vi "Remove Units Panel 2.vi"(0 "System#":u8, 7 "Rack Number":i8=2 min=1 max=16, 8 "AutoAge.ini  File Path":path=path "\\\\Beco\\autoage/config/autoage.ini") -> ()   [LabVIEW 2021]
uses:
  Main Controls System v8.0/AutoAge Globals.vi
panel:
  in  "Update":bool
  in  "Row33 to 40":bool
  in  "Row25 to 32":bool
  in  "Row17 to 24":bool
  in  "Row9 to 16":bool
  in  "Row1 to 8":bool
  in  "Select All":bool
  in  "40":bool
  in  "39":bool
  in  "38":bool
  in  "37":bool
  in  "36":bool
  in  "35":bool
  in  "34":bool
  in  "33":bool
  in  "32":bool
  in  "31":bool
  in  "30":bool
  in  "29":bool
  in  "28":bool
  in  "27":bool
  in  "26":bool
  in  "25":bool
  in  "24":bool
  in  "23":bool
  in  "22":bool
  in  "21":bool
  in  "20":bool
  in  "19":bool
  in  "18":bool
  in  "17":bool
  in  "16":bool
  in  "15":bool
  in  "14":bool
  in  "13":bool
  in  "12":bool
  in  "11":bool
  in  "10":bool
  in  "9":bool
  in  "8":bool
  in  "7":bool
  in  "6":bool
  in  "5":bool
  in  "4":bool
  in  "3":bool
  in  "2":bool
  in  "1":bool
  out "Rack":i8=1 min=1 max=16
  in  "Done":bool
  # "Click to Remove active positions.  A red square in a position indicates that a position is going to run."
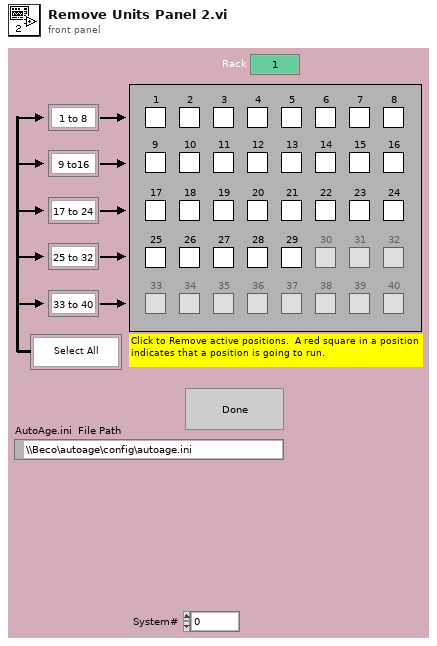
[diagram p1: front panel]
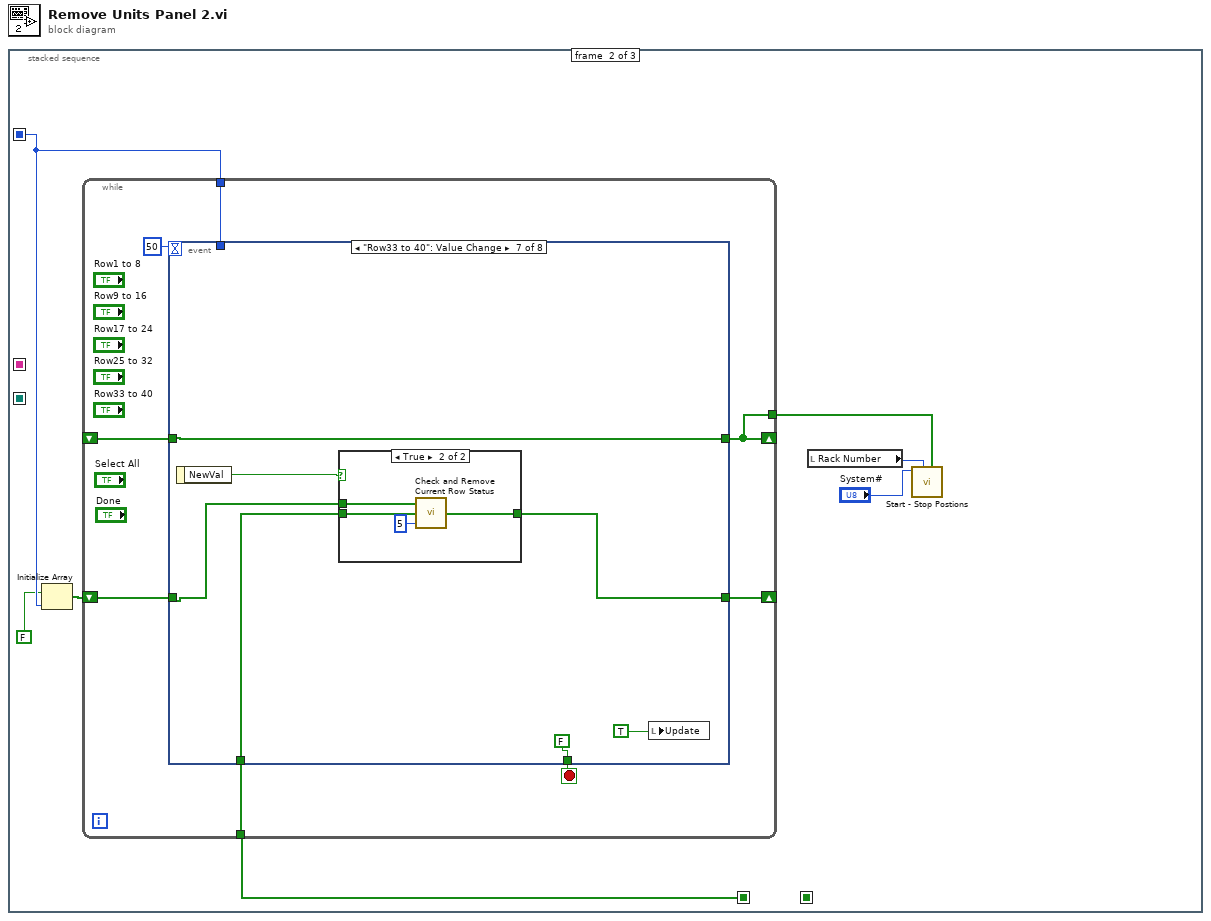
[diagram p0: block diagram]
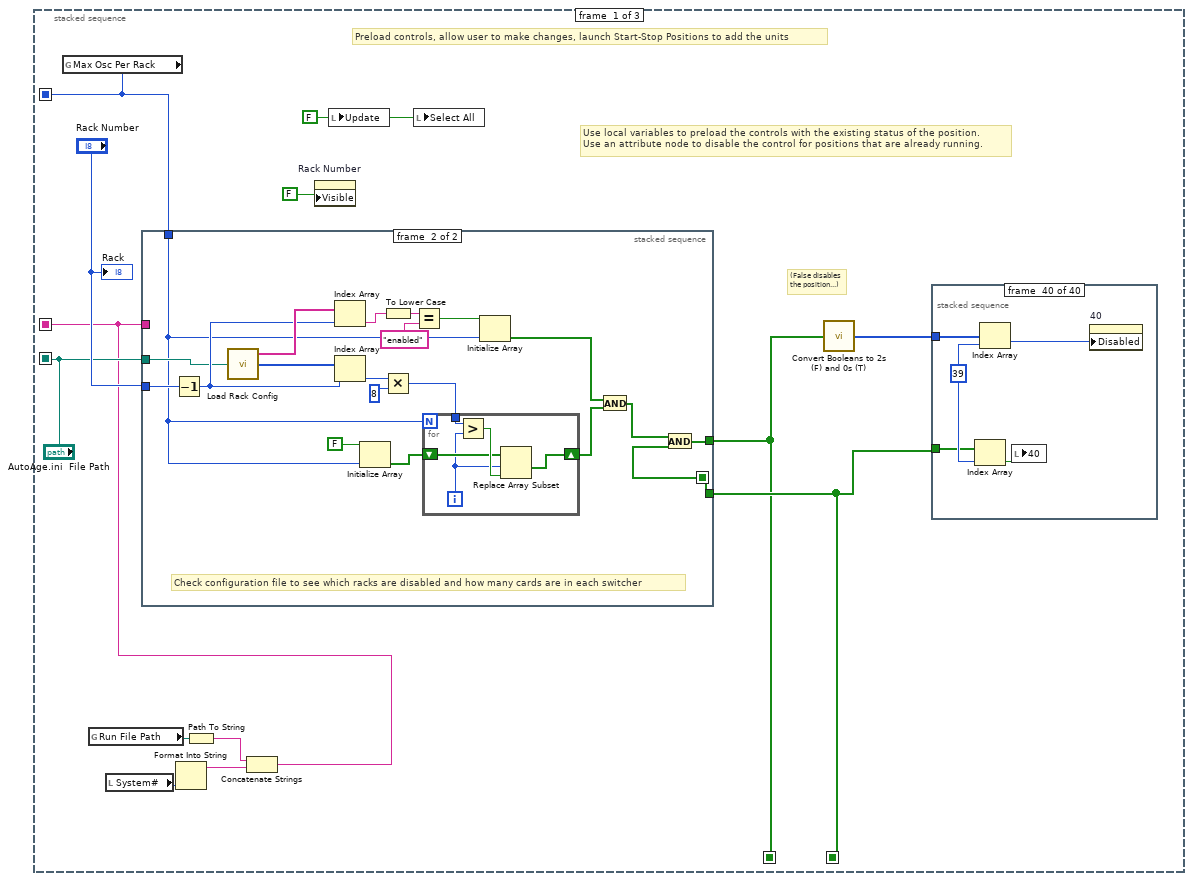
[diagram p2: hidden frame]
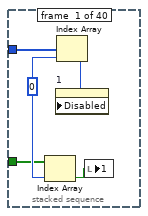
[diagram p3: hidden frame]
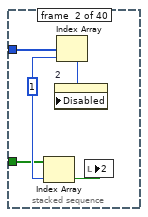
[diagram p4: hidden frame]
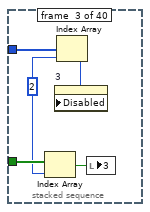
[diagram p5: hidden frame]
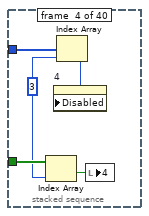
[diagram p6: hidden frame]
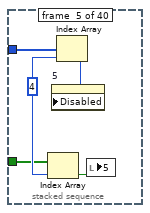
[diagram p7: hidden frame]
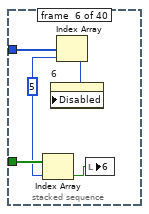
[diagram p8: hidden frame]
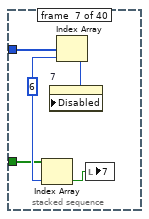
[diagram p9: hidden frame]
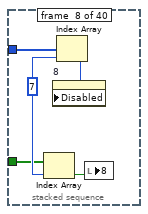
[diagram p10: hidden frame]
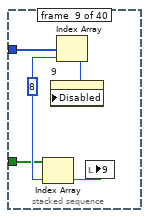
[diagram p11: hidden frame]
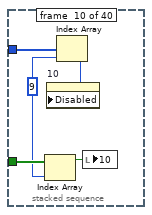
[diagram p12: hidden frame]
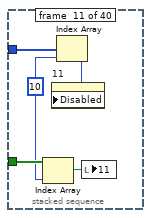
[diagram p13: hidden frame]
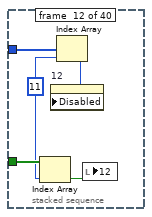
[diagram p14: hidden frame]
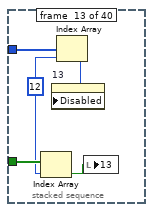
[diagram p15: hidden frame]
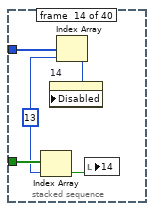
[diagram p16: hidden frame]
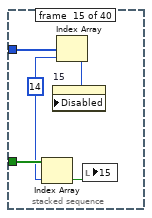
[diagram p17: hidden frame]
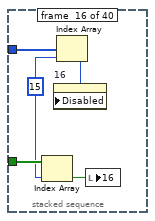
[diagram p18: hidden frame]
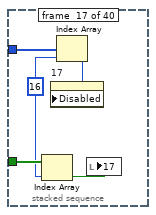
[diagram p19: hidden frame]
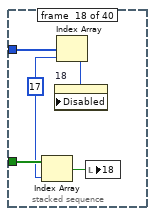
[diagram p20: hidden frame]
diagram:
  n1 = stacked-sequence {
    seq-local: [w10 _ _] -> [_ _ _]
    seq-local: [w9 _ _] -> [_ w267 _]
    seq-local: [w7 _ _] -> [_ w266 _]
    seq-local: ["AutoAge.ini  File Path" _ _] -> [_ _ _]
    seq-local: [w1 _ _] -> [_ _ _]
    frame #0 {
      w8 = FALSE ("Update")
      # "(False disables\nthe position...)"
      # "Preload controls, allow user to make changes, launch Start-Stop Positions to add the units"
      # "Use local variables to preload the controls with the existing status of the position.\nUse an attribute node to disable the control for positions that are already running."
      n2 = global read "AutoAge Globals.vi" "Max Osc Per Rack"() -> (w7:u16)
      n3 = global read "AutoAge Globals.vi" "Run File Path"() -> (w3:path)
      n4 = local read "System#"() -> (w4:u8)
      n5 = Format Into String(w4) -> (resulting string=w6:string)  [unwired: 3 in, 1 out]
      n6 = Path To String(path=w3) -> (string=w5:string)
      n7 = Concatenate Strings(w5, w6) -> (w1:string)
      n8 = stacked-sequence {
        seq-local: [w217 _] -> [_ w242]
        tunnel: "Rack Number" -> [w216 w250]
        tunnel: [_ w241] -> w9
        tunnel: [_ w242] -> w10
        tunnel: "AutoAge.ini  File Path" -> [_ w239]
        tunnel: w1 -> [w215 _]
        tunnel: w7 -> [w214 w238]
        frame #0 {
          # "Scan the disk to see which positions are currently running"
          n9 = for {
            N: w214 -> [_]
            tunnel: [w235] -> w217 mode=indexing
            tunnel: w216 -> [w223]
            tunnel: w215 -> [w220]
            i -> [w236]
            w221 = "-"
            n10 = Increment(x=w236) -> (x+1=w224:i32)
            n11 = Number To Decimal String(number=w223) -> (decimal integer string=w227:string)  [unwired: 1 in]
            n12 = Number To Decimal String(number=w224) -> (decimal integer string=w226:string)  [unwired: 1 in]
            n13 = Concatenate Strings(w220, w221, w227, w221, w226, ".run") -> (w225:string)
            n14 = String To Path(string=w225) -> (path=w234:path)
            n15 = Open/Create/Replace File(file path (use dialog)=w234, access (0:read/write)=1) -> (refnum out=w218:refnum<file>, error out=w219:errorcluster)  [unwired: 4 in, 1 out]
            n16 = Deny Access(4:w219, 6:1, 7:w218) -> (0:w231:errorcluster, 3:w228:refnum<file>)
            n17 = Close File(refnum=w228) -> ()  [unwired: 1 in, 2 out]
            n18 = Unbundle(w231) -> ("code"=w229:i32)  [unwired: 2 out]
            n19 = Equal?(x=w229, y=0) -> (x = y?=w235:bool)
          }
        }
        frame #1 {
          # "Check configuration file to see which racks are disabled and how many cards are in each switcher"
          n20 = Decrement(x=w250) -> (x-1=w240:i8)
          n21 = call "Load Rack Config"("AutoAge.ini  File Path"=w239) -> ("Rack Status"=w251:string[], "# of Cards"=w255:i32[])  [unwired: 1 out]
          n22 = Index Array(array=w251, index=w240) -> (element=w249:string)
          n23 = Index Array(array=w255, index=w240) -> (element=w256:i32)
          n24 = Initialize Array(FALSE, w238) -> (w245:bool[])
          n25 = To Lower Case(string=w249) -> (all lower case string=w254:string)
          n26 = Multiply(x=w256, y=8) -> (x*y=w246:i32)
          n27 = Equal?(x=w254, y="enabled") -> (x = y?=w248:bool)
          n28 = for {
            N: w238 -> [_]
            tunnel: w246 -> [w261]
            shift-right: [w258] -> w243
            shift-left: w245 -> [w259]
            i -> [w257]
            n29 = Greater?(x=w261, y=w257) -> (0:w260:bool)
            n30 = Replace Array Subset(array=w259, new element=w260, index=w257) -> (w258:bool[])
          }
          n31 = Initialize Array(w248, w238) -> (w244:bool[])
          n32 = And(x=w244, y=w243) -> (x .and. y?=w237:bool[])
          n33 = And(x=w237, y=w242) -> (x .and. y?=w241:bool[])
        }
      }
      n34 = property on="Rack Number" class="DigNum (strict)"("Visible"=FALSE) -> ()  [unwired: 2 in, 2 out]
      n35 = local write "Update"(w8) -> ()
      n36 = local write "Select All"(w8) -> ()
      n37 = call "Convert Booleans to 2s (F) and 0s (T)"("Boolean Array"=w9) -> ("2s and 0s"=w11:i8[])
      n38 = stacked-sequence {
        tunnel: w11 -> [w18 w23 w28 w33 w38 w43 w48 w53 w58 w63 w68 w73 w78 w83 w88 w93 w98 w103 w108 w113 w118 w123 w128 w133 w138 w143 w148 w153 w158 w163 w168 w173 w178 w183 w188 w193 w198 w203 w208 w213]
        tunnel: w10 -> [w15 w20 w27 w32 w36 w42 w46 w51 w56 w62 w67 w72 w77 w82 w87 w92 w97 w102 w107 w112 w117 w122 w127 w132 w137 w142 w147 w152 w157 w162 w167 w172 w177 w182 w187 w192 w197 w202 w207 w210]
        frame #0 {
          w16 = 0
          n39 = Index Array(array=w15, index=w16) -> (element=w17:bool)
          n40 = Index Array(array=w18, index=w16) -> (element=w14:i8)
          n41 = property on="1" class="Bool (strict)"("Disabled"=w14) -> ()  [unwired: 2 in, 2 out]
          n42 = local write "1"(w17) -> ()
        }
        frame #1 {
          w22 = 1
          n43 = Index Array(array=w20, index=w22) -> (element=w21:bool)
          n44 = Index Array(array=w23, index=w22) -> (element=w19:i8)
          n45 = property on="2" class="Bool (strict)"("Disabled"=w19) -> ()  [unwired: 2 in, 2 out]
          n46 = local write "2"(w21) -> ()
        }
        frame #2 {
          w26 = 2
          n47 = Index Array(array=w27, index=w26) -> (element=w25:bool)
          n48 = Index Array(array=w28, index=w26) -> (element=w24:i8)
          n49 = property on="3" class="Bool (strict)"("Disabled"=w24) -> ()  [unwired: 2 in, 2 out]
          n50 = local write "3"(w25) -> ()
        }
        frame #3 {
          w31 = 3
          n51 = Index Array(array=w32, index=w31) -> (element=w30:bool)
          n52 = Index Array(array=w33, index=w31) -> (element=w29:i8)
          n53 = property on="4" class="Bool (strict)"("Disabled"=w29) -> ()  [unwired: 2 in, 2 out]
          n54 = local write "4"(w30) -> ()
        }
        frame #4 {
          w37 = 4
          n55 = Index Array(array=w36, index=w37) -> (element=w35:bool)
          n56 = Index Array(array=w38, index=w37) -> (element=w34:i8)
          n57 = property on="5" class="Bool (strict)"("Disabled"=w34) -> ()  [unwired: 2 in, 2 out]
          n58 = local write "5"(w35) -> ()
        }
        frame #5 {
          w41 = 5
          n59 = Index Array(array=w42, index=w41) -> (element=w40:bool)
          n60 = Index Array(array=w43, index=w41) -> (element=w39:i8)
          n61 = property on="6" class="Bool (strict)"("Disabled"=w39) -> ()  [unwired: 2 in, 2 out]
          n62 = local write "6"(w40) -> ()
        }
        frame #6 {
          w47 = 6
          n63 = Index Array(array=w46, index=w47) -> (element=w45:bool)
          n64 = Index Array(array=w48, index=w47) -> (element=w44:i8)
          n65 = property on="7" class="Bool (strict)"("Disabled"=w44) -> ()  [unwired: 2 in, 2 out]
          n66 = local write "7"(w45) -> ()
        }
        frame #7 {
          w52 = 7
          n67 = Index Array(array=w51, index=w52) -> (element=w50:bool)
          n68 = Index Array(array=w53, index=w52) -> (element=w49:i8)
          n69 = property on="8" class="Bool (strict)"("Disabled"=w49) -> ()  [unwired: 2 in, 2 out]
          n70 = local write "8"(w50) -> ()
        }
        frame #8 {
          w57 = 8
          n71 = Index Array(array=w56, index=w57) -> (element=w55:bool)
          n72 = Index Array(array=w58, index=w57) -> (element=w54:i8)
          n73 = property on="9" class="Bool (strict)"("Disabled"=w54) -> ()  [unwired: 2 in, 2 out]
          n74 = local write "9"(w55) -> ()
        }
        frame #9 {
          w60 = 9
          n75 = Index Array(array=w62, index=w60) -> (element=w61:bool)
          n76 = Index Array(array=w63, index=w60) -> (element=w59:i8)
          n77 = property on="10" class="Bool (strict)"("Disabled"=w59) -> ()  [unwired: 2 in, 2 out]
          n78 = local write "10"(w61) -> ()
        }
        frame #10 {
          w65 = 10
          n79 = Index Array(array=w67, index=w65) -> (element=w66:bool)
          n80 = Index Array(array=w68, index=w65) -> (element=w64:i8)
          n81 = property on="11" class="Bool (strict)"("Disabled"=w64) -> ()  [unwired: 2 in, 2 out]
          n82 = local write "11"(w66) -> ()
        }
        frame #11 {
          w70 = 11
          n83 = Index Array(array=w72, index=w70) -> (element=w71:bool)
          n84 = Index Array(array=w73, index=w70) -> (element=w69:i8)
          n85 = property on="12" class="Bool (strict)"("Disabled"=w69) -> ()  [unwired: 2 in, 2 out]
          n86 = local write "12"(w71) -> ()
        }
        frame #12 {
          w75 = 12
          n87 = Index Array(array=w77, index=w75) -> (element=w76:bool)
          n88 = Index Array(array=w78, index=w75) -> (element=w74:i8)
          n89 = property on="13" class="Bool (strict)"("Disabled"=w74) -> ()  [unwired: 2 in, 2 out]
          n90 = local write "13"(w76) -> ()
        }
        frame #13 {
          w81 = 13
          n91 = Index Array(array=w82, index=w81) -> (element=w80:bool)
          n92 = Index Array(array=w83, index=w81) -> (element=w79:i8)
          n93 = property on="14" class="Bool (strict)"("Disabled"=w79) -> ()  [unwired: 2 in, 2 out]
          n94 = local write "14"(w80) -> ()
        }
        frame #14 {
          w86 = 14
          n95 = Index Array(array=w87, index=w86) -> (element=w85:bool)
          n96 = Index Array(array=w88, index=w86) -> (element=w84:i8)
          n97 = property on="15" class="Bool (strict)"("Disabled"=w84) -> ()  [unwired: 2 in, 2 out]
          n98 = local write "15"(w85) -> ()
        }
        frame #15 {
          w91 = 15
          n99 = Index Array(array=w92, index=w91) -> (element=w90:bool)
          n100 = Index Array(array=w93, index=w91) -> (element=w89:i8)
          n101 = property on="16" class="Bool (strict)"("Disabled"=w89) -> ()  [unwired: 2 in, 2 out]
          n102 = local write "16"(w90) -> ()
        }
        frame #16 {
          w96 = 16
          n103 = Index Array(array=w97, index=w96) -> (element=w95:bool)
          n104 = Index Array(array=w98, index=w96) -> (element=w94:i8)
          n105 = property on="17" class="Bool (strict)"("Disabled"=w94) -> ()  [unwired: 2 in, 2 out]
          n106 = local write "17"(w95) -> ()
        }
        frame #17 {
          w101 = 17
          n107 = Index Array(array=w102, index=w101) -> (element=w100:bool)
          n108 = Index Array(array=w103, index=w101) -> (element=w99:i8)
          n109 = property on="18" class="Bool (strict)"("Disabled"=w99) -> ()  [unwired: 2 in, 2 out]
          n110 = local write "18"(w100) -> ()
        }
        frame #18 {
          w106 = 18
          n111 = Index Array(array=w107, index=w106) -> (element=w105:bool)
          n112 = Index Array(array=w108, index=w106) -> (element=w104:i8)
          n113 = property on="19" class="Bool (strict)"("Disabled"=w104) -> ()  [unwired: 2 in, 2 out]
          n114 = local write "19"(w105) -> ()
        }
        frame #19 {
          w111 = 19
          n115 = Index Array(array=w112, index=w111) -> (element=w110:bool)
          n116 = Index Array(array=w113, index=w111) -> (element=w109:i8)
          n117 = property on="20" class="Bool (strict)"("Disabled"=w109) -> ()  [unwired: 2 in, 2 out]
          n118 = local write "20"(w110) -> ()
        }
        frame #20 {
          w115 = 20
          n119 = Index Array(array=w117, index=w115) -> (element=w116:bool)
          n120 = Index Array(array=w118, index=w115) -> (element=w114:i8)
          n121 = property on="21" class="Bool (strict)"("Disabled"=w114) -> ()  [unwired: 2 in, 2 out]
          n122 = local write "21"(w116) -> ()
        }
        frame #21 {
          w121 = 21
          n123 = Index Array(array=w122, index=w121) -> (element=w120:bool)
          n124 = Index Array(array=w123, index=w121) -> (element=w119:i8)
          n125 = property on="22" class="Bool (strict)"("Disabled"=w119) -> ()  [unwired: 2 in, 2 out]
          n126 = local write "22"(w120) -> ()
        }
        frame #22 {
          w126 = 22
          n127 = Index Array(array=w127, index=w126) -> (element=w125:bool)
          n128 = Index Array(array=w128, index=w126) -> (element=w124:i8)
          n129 = property on="23" class="Bool (strict)"("Disabled"=w124) -> ()  [unwired: 2 in, 2 out]
          n130 = local write "23"(w125) -> ()
        }
        frame #23 {
          w131 = 23
          n131 = Index Array(array=w132, index=w131) -> (element=w130:bool)
          n132 = Index Array(array=w133, index=w131) -> (element=w129:i8)
          n133 = property on="24" class="Bool (strict)"("Disabled"=w129) -> ()  [unwired: 2 in, 2 out]
          n134 = local write "24"(w130) -> ()
        }
        frame #24 {
          w136 = 24
          n135 = Index Array(array=w137, index=w136) -> (element=w135:bool)
          n136 = Index Array(array=w138, index=w136) -> (element=w134:i8)
          n137 = property on="25" class="Bool (strict)"("Disabled"=w134) -> ()  [unwired: 2 in, 2 out]
          n138 = local write "25"(w135) -> ()
        }
        frame #25 {
          w141 = 25
          n139 = Index Array(array=w142, index=w141) -> (element=w140:bool)
          n140 = Index Array(array=w143, index=w141) -> (element=w139:i8)
          n141 = property on="26" class="Bool (strict)"("Disabled"=w139) -> ()  [unwired: 2 in, 2 out]
          n142 = local write "26"(w140) -> ()
        }
        frame #26 {
          w146 = 26
          n143 = Index Array(array=w147, index=w146) -> (element=w145:bool)
          n144 = Index Array(array=w148, index=w146) -> (element=w144:i8)
          n145 = property on="27" class="Bool (strict)"("Disabled"=w144) -> ()  [unwired: 2 in, 2 out]
          n146 = local write "27"(w145) -> ()
        }
        frame #27 {
          w151 = 27
          n147 = Index Array(array=w152, index=w151) -> (element=w150:bool)
          n148 = Index Array(array=w153, index=w151) -> (element=w149:i8)
          n149 = property on="28" class="Bool (strict)"("Disabled"=w149) -> ()  [unwired: 2 in, 2 out]
          n150 = local write "28"(w150) -> ()
        }
        frame #28 {
          w156 = 28
          n151 = Index Array(array=w157, index=w156) -> (element=w155:bool)
          n152 = Index Array(array=w158, index=w156) -> (element=w154:i8)
          n153 = property on="29" class="Bool (strict)"("Disabled"=w154) -> ()  [unwired: 2 in, 2 out]
          n154 = local write "29"(w155) -> ()
        }
        frame #29 {
          w161 = 29
          n155 = Index Array(array=w162, index=w161) -> (element=w160:bool)
          n156 = Index Array(array=w163, index=w161) -> (element=w159:i8)
          n157 = property on="30" class="Bool (strict)"("Disabled"=w159) -> ()  [unwired: 2 in, 2 out]
          n158 = local write "30"(w160) -> ()
        }
        frame #30 {
          w166 = 30
          n159 = Index Array(array=w167, index=w166) -> (element=w165:bool)
          n160 = Index Array(array=w168, index=w166) -> (element=w164:i8)
          n161 = property on="31" class="Bool (strict)"("Disabled"=w164) -> ()  [unwired: 2 in, 2 out]
          n162 = local write "31"(w165) -> ()
        }
        frame #31 {
          w171 = 31
          n163 = Index Array(array=w172, index=w171) -> (element=w170:bool)
          n164 = Index Array(array=w173, index=w171) -> (element=w169:i8)
          n165 = property on="32" class="Bool (strict)"("Disabled"=w169) -> ()  [unwired: 2 in, 2 out]
          n166 = local write "32"(w170) -> ()
        }
        frame #32 {
          w176 = 32
          n167 = Index Array(array=w177, index=w176) -> (element=w175:bool)
          n168 = Index Array(array=w178, index=w176) -> (element=w174:i8)
          n169 = property on="33" class="Bool (strict)"("Disabled"=w174) -> ()  [unwired: 2 in, 2 out]
          n170 = local write "33"(w175) -> ()
        }
        frame #33 {
          w181 = 33
          n171 = Index Array(array=w182, index=w181) -> (element=w180:bool)
          n172 = Index Array(array=w183, index=w181) -> (element=w179:i8)
          n173 = property on="34" class="Bool (strict)"("Disabled"=w179) -> ()  [unwired: 2 in, 2 out]
          n174 = local write "34"(w180) -> ()
        }
        frame #34 {
          w186 = 34
          n175 = Index Array(array=w187, index=w186) -> (element=w185:bool)
          n176 = Index Array(array=w188, index=w186) -> (element=w184:i8)
          n177 = property on="35" class="Bool (strict)"("Disabled"=w184) -> ()  [unwired: 2 in, 2 out]
          n178 = local write "35"(w185) -> ()
        }
        frame #35 {
          w191 = 35
          n179 = Index Array(array=w192, index=w191) -> (element=w190:bool)
          n180 = Index Array(array=w193, index=w191) -> (element=w189:i8)
          n181 = property on="36" class="Bool (strict)"("Disabled"=w189) -> ()  [unwired: 2 in, 2 out]
          n182 = local write "36"(w190) -> ()
        }
        frame #36 {
          w196 = 36
          n183 = Index Array(array=w197, index=w196) -> (element=w195:bool)
          n184 = Index Array(array=w198, index=w196) -> (element=w194:i8)
          n185 = property on="37" class="Bool (strict)"("Disabled"=w194) -> ()  [unwired: 2 in, 2 out]
          n186 = local write "37"(w195) -> ()
        }
        frame #37 {
          w201 = 37
          n187 = Index Array(array=w202, index=w201) -> (element=w200:bool)
          n188 = Index Array(array=w203, index=w201) -> (element=w199:i8)
          n189 = property on="38" class="Bool (strict)"("Disabled"=w199) -> ()  [unwired: 2 in, 2 out]
          n190 = local write "38"(w200) -> ()
        }
        frame #38 {
          w206 = 38
          n191 = Index Array(array=w207, index=w206) -> (element=w205:bool)
          n192 = Index Array(array=w208, index=w206) -> (element=w204:i8)
          n193 = property on="39" class="Bool (strict)"("Disabled"=w204) -> ()  [unwired: 2 in, 2 out]
          n194 = local write "39"(w205) -> ()
        }
        frame #39 {
          w211 = 39
          n195 = Index Array(array=w210, index=w211) -> (element=w212:bool)
          n196 = Index Array(array=w213, index=w211) -> (element=w209:i8)
          n197 = local write "40"(w212) -> ()
          n198 = property on="40" class="Bool (strict)"("Disabled"=w209) -> ()  [unwired: 2 in, 2 out]
        }
      }
      "Rack" <- "Rack Number"
    }
    frame #1 {
      n199 = Initialize Array(FALSE, w266) -> (w264:bool[])
      n200 = while {
        tunnel: w267 -> [w274]
        tunnel: w266 -> [w275]
        shift-right: [w269] -> _
        shift-left: _ -> [w272]
        shift-right: [w270] -> _
        shift-left: w264 -> [w271]
        tunnel: [w269] -> w268
        stop <- w273 stop-if-true
        n201 = event shown="[6] \"Row33 to 40\": Value Change" {
          selector: _ -> [_ _ _ _ _ _ _ _]
          dyn-events: _ -> [_ _ _ _ _ _ _ _]
          timeout: 50 -> [_ _ _ _ _ _ _ _]
          tunnel: w275 -> [w280 _ _ _ _ _ _ w436]
          tunnel: w274 -> [w277 _ w377 w389 w401 w413 w425 w439]
          tunnel: [FALSE w374 FALSE ("NewVal") FALSE ("NewVal") FALSE ("NewVal") FALSE ("NewVal") FALSE ("NewVal") FALSE ("NewVal")] -> w273
          tunnel: w272 -> [_ w373 w375 w387 w399 w411 w423 w435]
          tunnel: w271 -> [w279 _ w378 w390 w402 w414 w426 w438]
          tunnel: [w278 _ w376 w388 w400 w412 w424 w437] -> w270
          tunnel: [w278 w373 w375 w387 w399 w411 w423 w435] -> w269
          event Timeout {
            n202 = event-data() -> ()  [unwired: 1 in, 1 out]
            n203 = case shown="True" "Update" {
              tunnel: [w323 w324] -> w278
              tunnel: w280 -> [_ w328]
              tunnel: w279 -> [_ w327]
              tunnel: w277 -> [_ w326]
              frame False {
                # "The actual controls"
                n204 = Build Array("1", "2", "3", "4", "5", "6", "7", "8", "9", "10", "11", "12", "13", "14", "15", "16", "17", "18", "19", "20", "21", "22", "23", "24", "25", "26", "27", "28", "29", "30", "31", "32", "33", "34", "35", "36", "37", "38", "39", "40") -> (w323:bool[])
              }
              frame True {
                n205 = for {
                  N: w328 -> [_]
                  tunnel: w327 -> [w331] mode=indexing
                  tunnel: w326 -> [w329] mode=indexing
                  tunnel: [w330] -> w324 mode=indexing
                  i -> [w332]
                  n206 = And(x=w329, y=w331) -> (x .and. y?=w330:bool)
                  n207 = case shown="0, Default" w332 {
                    tunnel: w330 -> [w333 w334 w335 w336 w337 w338 w339 w340 w341 w342 w343 w344 w345 w346 w347 w348 w349 w350 w351 w352 w353 w354 w355 w356 w357 w358 w359 w360 w361 w362 w363 w364 w365 w366 w367 w368 w369 w370 w371 w372]
                    frame 0, Default {
                      n208 = local write "1"(w333) -> ()
                    }
                    frame 1 {
                      n209 = local write "2"(w334) -> ()
                    }
                    frame 2 {
                      n210 = local write "3"(w335) -> ()
                    }
                    frame 3 {
                      n211 = local write "4"(w336) -> ()
                    }
                    frame 4 {
                      n212 = local write "5"(w337) -> ()
                    }
                    frame 5 {
                      n213 = local write "6"(w338) -> ()
                    }
                    frame 6 {
                      n214 = local write "7"(w339) -> ()
                    }
                    frame 7 {
                      n215 = local write "8"(w340) -> ()
                    }
                    frame 8 {
                      n216 = local write "9"(w341) -> ()
                    }
                    frame 9 {
                      n217 = local write "10"(w342) -> ()
                    }
                    frame 10 {
                      n218 = local write "11"(w343) -> ()
                    }
                    frame 11 {
                      n219 = local write "12"(w344) -> ()
                    }
                    frame 12 {
                      n220 = local write "13"(w345) -> ()
                    }
                    frame 13 {
                      n221 = local write "14"(w346) -> ()
                    }
                    frame 14 {
                      n222 = local write "15"(w347) -> ()
                    }
                    frame 15 {
                      n223 = local write "16"(w348) -> ()
                    }
                    frame 16 {
                      n224 = local write "17"(w349) -> ()
                    }
                    frame 17 {
                      n225 = local write "18"(w350) -> ()
                    }
                    frame 18 {
                      n226 = local write "19"(w351) -> ()
                    }
                    frame 19 {
                      n227 = local write "20"(w352) -> ()
                    }
                    frame 20 {
                      n228 = local write "21"(w353) -> ()
                    }
                    frame 21 {
                      n229 = local write "22"(w354) -> ()
                    }
                    frame 22 {
                      n230 = local write "23"(w355) -> ()
                    }
                    frame 23 {
                      n231 = local write "24"(w356) -> ()
                    }
                    frame 24 {
                      n232 = local write "25"(w357) -> ()
                    }
                    frame 25 {
                      n233 = local write "26"(w358) -> ()
                    }
                    frame 26 {
                      n234 = local write "27"(w359) -> ()
                    }
                    frame 27 {
                      n235 = local write "28"(w360) -> ()
                    }
                    frame 28 {
                      n236 = local write "29"(w361) -> ()
                    }
                    frame 29 {
                      n237 = local write "30"(w362) -> ()
                    }
                    frame 30 {
                      n238 = local write "31"(w363) -> ()
                    }
                    frame 31 {
                      n239 = local write "32"(w364) -> ()
                    }
                    frame 32 {
                      n240 = local write "33"(w365) -> ()
                    }
                    frame 33 {
                      n241 = local write "34"(w366) -> ()
                    }
                    frame 34 {
                      n242 = local write "35"(w367) -> ()
                    }
                    frame 35 {
                      n243 = local write "36"(w368) -> ()
                    }
                    frame 36 {
                      n244 = local write "37"(w369) -> ()
                    }
                    frame 37 {
                      n245 = local write "38"(w370) -> ()
                    }
                    frame 38 {
                      n246 = local write "39"(w371) -> ()
                    }
                    frame 39 {
                      n247 = local write "40"(w372) -> ()
                    }
                  }
                }
                n248 = local write "Update"(FALSE ("Update")) -> ()
              }
            }
          }
          event "Done": Value Change {
            n249 = event-data() -> ("NewVal"=w374:bool)  [unwired: 1 in]
          }
          event "Row1 to 8": Value Change {
            n250 = event-data() -> ("NewVal"=w379:bool)  [unwired: 1 in]
            n251 = case shown="True" w379 {
              tunnel: w377 -> [_ w385]
              tunnel: w378 -> [w382 w384]
              tunnel: [w382 w383] -> w376
              frame False {
              }
              frame True {
                n252 = call "Check and Remove Current Row Status.vi"("Row"=1, "Active Positions"=w385, "Rack Status In"=w384) -> ("Rack Status Out"=w383:bool[])
              }
            }
            n253 = local write "Update"(TRUE ("Update")) -> ()
          }
          event "Row9 to 16": Value Change {
            n254 = event-data() -> ("NewVal"=w391:bool)  [unwired: 1 in]
            n255 = case shown="True" w391 {
              tunnel: w389 -> [_ w397]
              tunnel: w390 -> [w394 w396]
              tunnel: [w394 w395] -> w388
              frame False {
              }
              frame True {
                n256 = call "Check and Remove Current Row Status.vi"("Row"=2, "Active Positions"=w397, "Rack Status In"=w396) -> ("Rack Status Out"=w395:bool[])
              }
            }
            n257 = local write "Update"(TRUE ("Update")) -> ()
          }
          event "Row17 to 24": Value Change {
            n258 = event-data() -> ("NewVal"=w403:bool)  [unwired: 1 in]
            n259 = case shown="True" w403 {
              tunnel: w401 -> [_ w409]
              tunnel: w402 -> [w406 w408]
              tunnel: [w406 w407] -> w400
              frame False {
              }
              frame True {
                n260 = call "Check and Remove Current Row Status.vi"("Row"=3, "Active Positions"=w409, "Rack Status In"=w408) -> ("Rack Status Out"=w407:bool[])
              }
            }
            n261 = local write "Update"(TRUE ("Update")) -> ()
          }
          event "Row25 to 32": Value Change {
            n262 = event-data() -> ("NewVal"=w415:bool)  [unwired: 1 in]
            n263 = case shown="True" w415 {
              tunnel: w413 -> [_ w421]
              tunnel: w414 -> [w418 w420]
              tunnel: [w418 w419] -> w412
              frame False {
              }
              frame True {
                n264 = call "Check and Remove Current Row Status.vi"("Row"=4, "Active Positions"=w421, "Rack Status In"=w420) -> ("Rack Status Out"=w419:bool[])
              }
            }
            n265 = local write "Update"(TRUE ("Update")) -> ()
          }
          event "Row33 to 40": Value Change {
            n266 = event-data() -> ("NewVal"=w427:bool)  [unwired: 1 in]
            n267 = case shown="True" w427 {
              tunnel: w425 -> [_ w433]
              tunnel: w426 -> [w430 w432]
              tunnel: [w430 w431] -> w424
              frame False {
              }
              frame True {
                n268 = call "Check and Remove Current Row Status.vi"("Row"=5, "Active Positions"=w433, "Rack Status In"=w432) -> ("Rack Status Out"=w431:bool[])
              }
            }
            n269 = local write "Update"(TRUE ("Update")) -> ()
          }
          event "Select All": Value Change {
            n270 = event-data() -> ("NewVal"=w440:bool)  [unwired: 1 in]
            n271 = case shown="True" w440 {
              tunnel: w439 -> [_ w445]
              tunnel: w438 -> [w443 w446]
              tunnel: [w443 w447] -> w437
              tunnel: w436 -> [_ w444]
              frame False {
              }
              frame True {
                n272 = call "Select All Positions for Curve Fit.vi"("Max Positions per Rack"=w444, "Rack Status In"=w446, "Active Positions"=w445) -> ("Rack Status Out"=w447:bool[])
              }
            }
            n273 = local write "Update"(TRUE ("Update")) -> ()
          }
        }
      }
      n274 = local read "Rack Number"() -> (w262:i8)
      n275 = call "Start - Stop Postions"("New Status of Positions"=w268, "Rack Number"=w262, "System#"="System#") -> ()  [unwired: 9 in]
    }
    frame #2 {
      # "Set \"Functional Test Required\" to TRUE so Data Acquistion will start the Auto Functional Check on the units just added"
      n276 = global write "Globals" "Functional Test Requested"(TRUE ("Functional Test Requested")) -> ()
    }
  }
